vi "globalSetUp.vi"(8 "error in (no error)":errorcluster, 11 "testcase-CSMArgument in":refnum<class "testcase-CSMArgument.lvclass">) -> (0 "error out":errorcluster, 3 "testcase-CSMArgument out":refnum<class "testcase-CSMArgument.lvclass">)   [LabVIEW 2017, in "testcase-CSMArgument.lvclass"]
uses:
  testcase-CSMArgument.lvclass
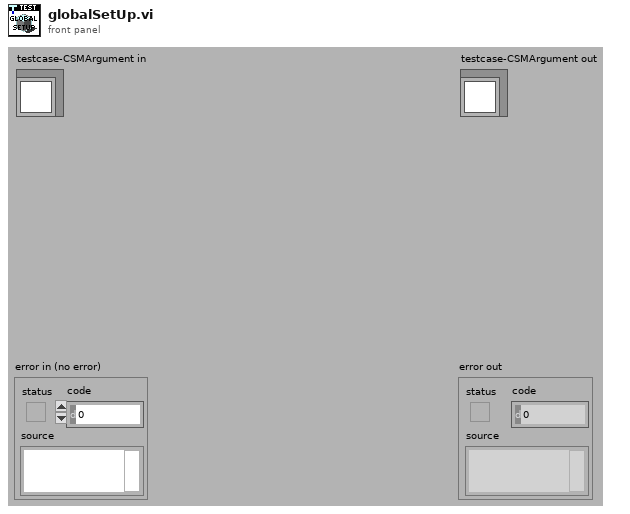
[diagram p1: front panel]
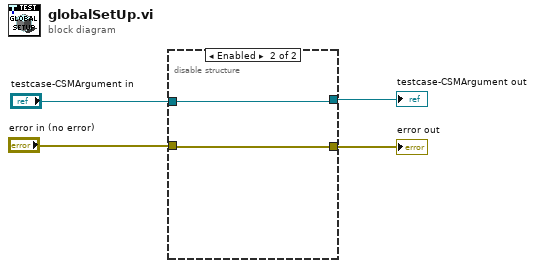
[diagram p0: block diagram]
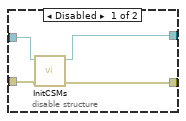
[diagram p2: hidden frame]
diagram:
  n1 = disable-structure shown="Enabled" {
    disable-tunnel: "testcase-CSMArgument in" -> [w8 w9]
    disable-tunnel: [w7 w9] -> w3
    disable-tunnel: "error in (no error)" -> [w6 w10]
    disable-tunnel: [w5 w10] -> w1
    frame Disabled {
      n2 = call "InitCSMs.vi"("error in"=w6, "testcase-CSMArgument.lvclass in"=w8) -> ("error out"=w5:errorcluster, "testcase-CSMArgument.lvclass out"=w7:refnum<class "testcase-CSMArgument.lvclass">)  [unwired: 8 in]
    }
    frame Enabled {
    }
  }
  "error out" <- w1
  "testcase-CSMArgument out" <- w3
